vi "Magnet Idot Monitor.vi"(8 "Error In":errorcluster, 10 "Server port":u16=1002, 11 "Server address":string="192.168.1.100") -> (0 "Error Out":errorcluster)   [LabVIEW 2015]
uses:
  Libraries/Red Pitaya/Mode.ctl
  Libraries/Red Pitaya/Red Pitaya Parameters.ctl
  Libraries/Red Pitaya/RP Command.ctl
  Libraries/Utilities/Controls/Integrate channel.ctl
panel:
  out "Magnet current":waveform(dbl)(graph)
  in  "Controls":enum32{"Basic", "Advanced"}(tab)
  in  "Idot \ncalibration":dbl=-137722.0
  in  "Parameters":T1={"Ranges"=[1.12291, 20.0], "Output frequency 1"=50000.0, "Output frequency 2"=50000.0, "Trigger offset"=-2000000, "Post-trigger samples"=5767168, "Desimation rate"=64} {"Post-trigger samples" format="0x%x (%d)"; "Trigger offset" format="0x%x (%d)"; "Output frequency 2" format="%#_6p"; "Output frequency 1" format="%#_6p"; "Ranges" format="%#_12g"}
  out "CPU Temperature":dbl(slide)=48.847186279148 scale=0.0..100.0
  out "Current min/max":cluster{"Max":dbl, "Min":dbl}
  in  "Offset duration":dbl=0.95
  in  "Ch to \nintegrate":i32
  in  "Trigger pos acuracy":i32=2
  in  "Signal bits":i32=16
  in  "Read Temperature":bool=TRUE
  in  "Read trigger":bool=TRUE
  in  "Start server":bool
  in  "FPGA Logic":enum16{"Digitizer", "Fast Digitizer"}(ring)
  in  "Auto-save file":bool=TRUE
  in  "Samples to read":u64=67108864 format="0x%x (%d)"
  in  "Record":bool
  out "Server  output":string
  out "Temperature Chart":dbl(graph)=48.847186279148
  out "bytes written":i32=8
  in  "Status":bool
  out "Status response":u32=1
  out "element":u32
  in  "Status offset":u64=8 format="%x"
  out "Record start pos":u32=1
  out "x-y":u32=4294967295
  out "Phase increment 2":u64=1717987
  out "Phase increment 1":u64=1717987
  in  "Process Stop Button":bool
  in  "Read":bool
  in  "Read subset":bool
  out "Data File  Path":path
  out "Trigger state":bool
  in  "Trigger":bool
  in  "Arm":bool
  out "Phase  Graph":u32[](graph)
  in  "Mode":T2=enum."Digitizer"
  out "Waveform Graph":sgl[][](graph)
  in  "Stop Server":bool
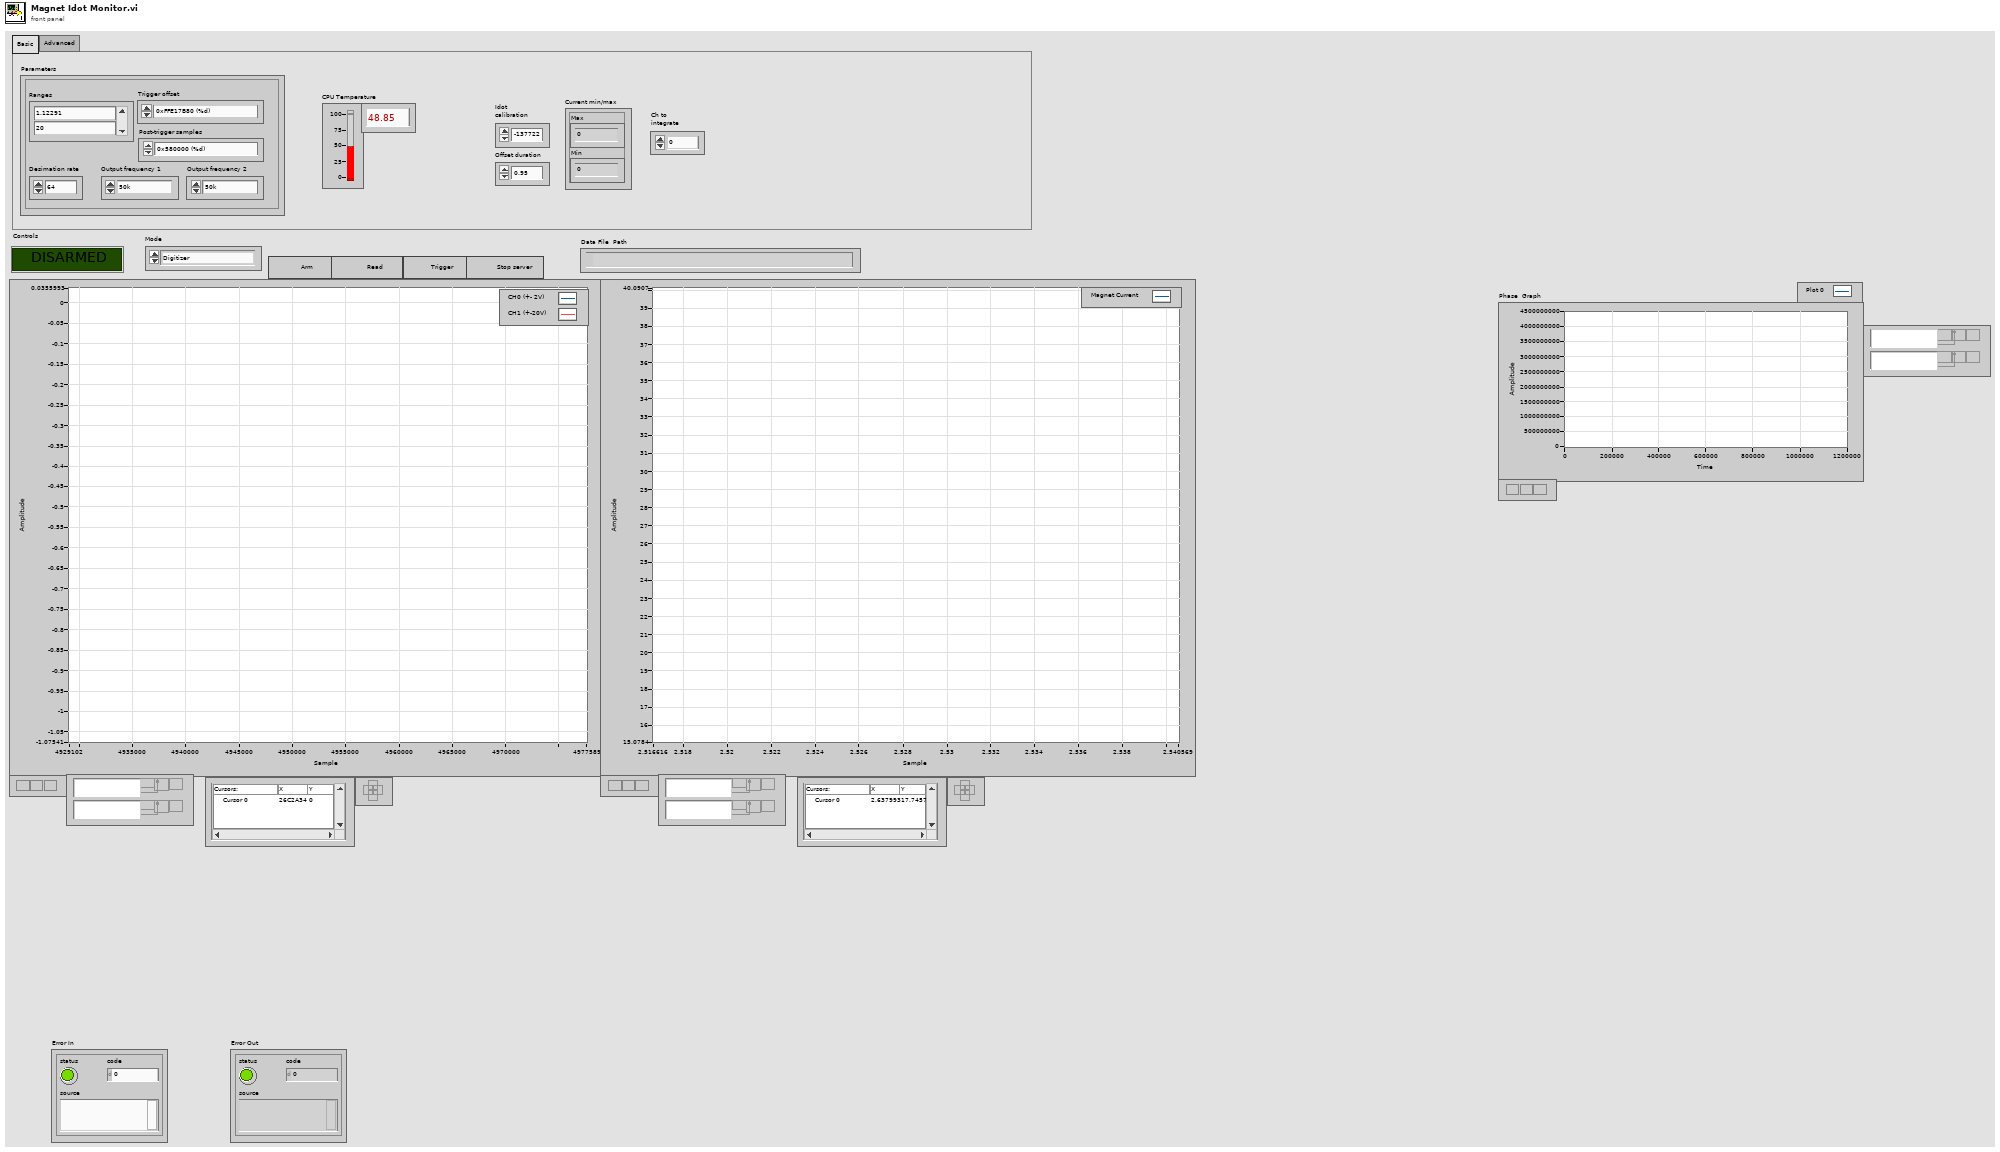
[diagram p1: front panel]
types:
  T1 = typedef "Red Pitaya Parameters.ctl" = cluster{"Ranges":dbl[], "Output frequency 1":dbl, "Output frequency 2":dbl, "Trigger offset":i32, "Post-trigger samples":u64, "Desimation rate":u64}
  T2 = typedef "Mode.ctl" = enum16{"Filter", "Lockin test", "Snapshot test", "Digitizer"}
  T3 = typedef "RP Command.ctl" = enum16{"Set frequency", "Arm and get data", "Stop server", "Get status", "Get temperature", "Set decimation", "Arm", "Software trigger", "Get whole buffer", "Get chunk", "System call", "Get config", "Set config"}
  T4 = typedef "Integrate channel.ctl" = cluster{"Channel":string, "Output name":string, "Factor":dbl, "Start time":dbl, "Duration":dbl}
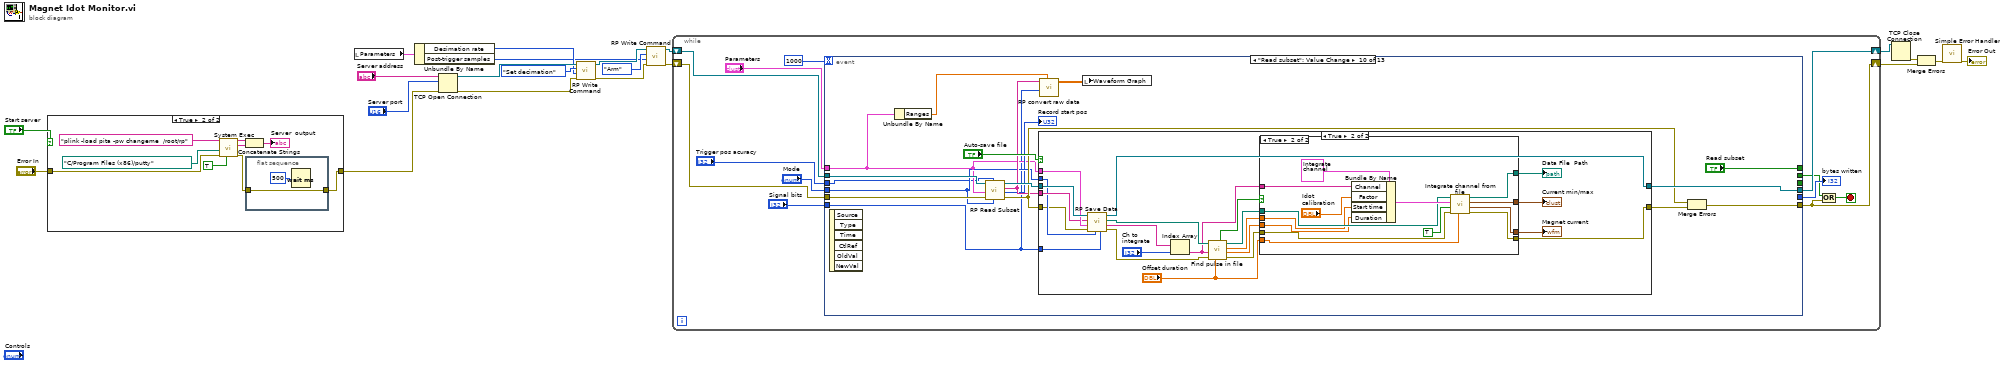
[diagram p0: block diagram]
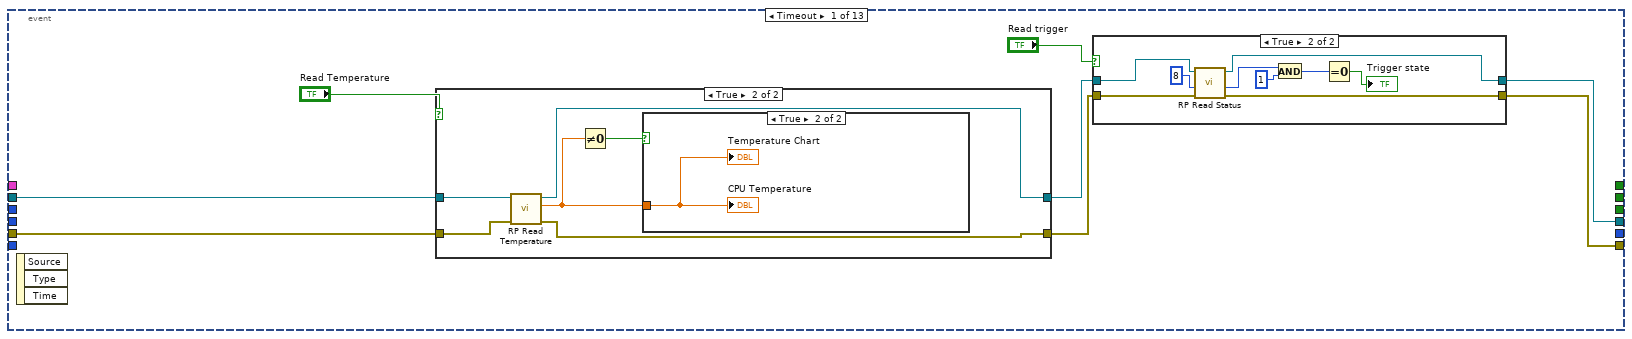
[diagram p3: hidden frame]
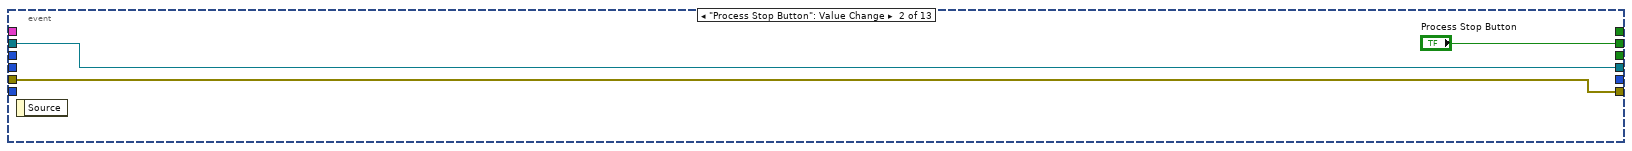
[diagram p7: hidden frame]
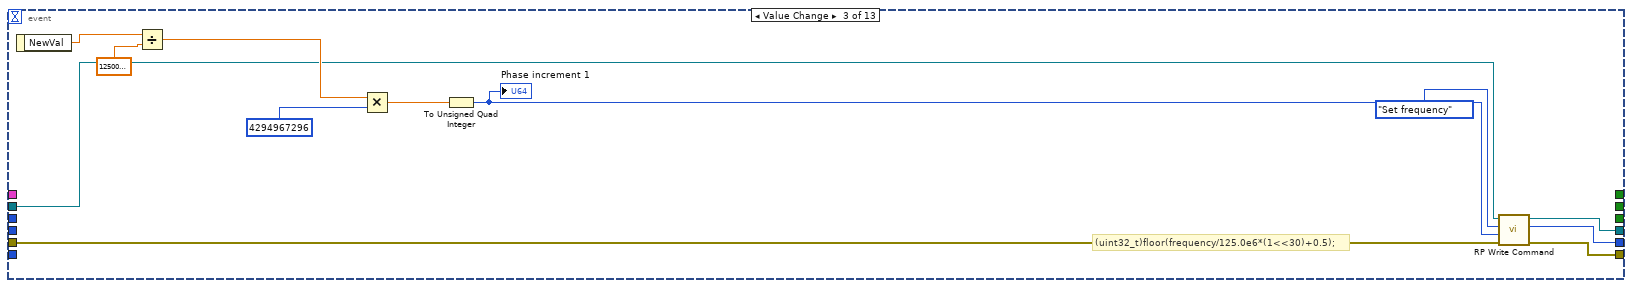
[diagram p8: hidden frame]
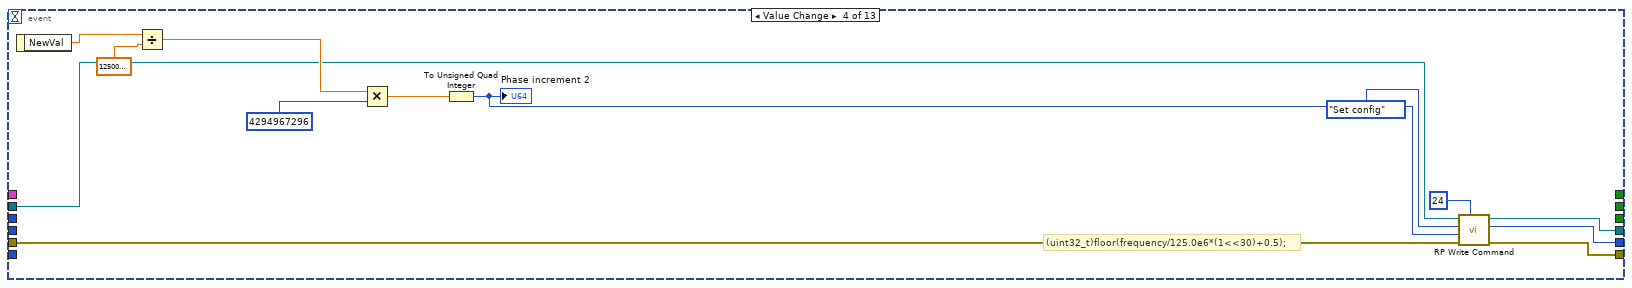
[diagram p9: hidden frame]
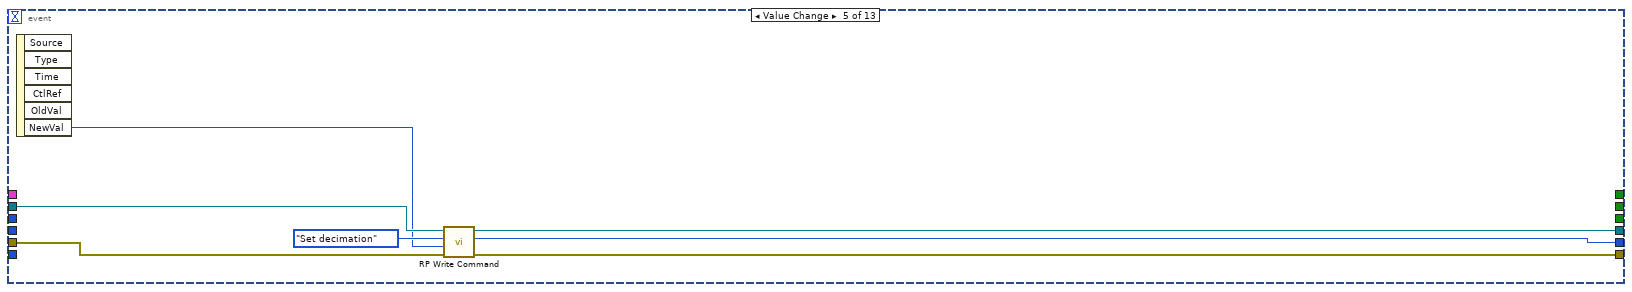
[diagram p10: hidden frame]
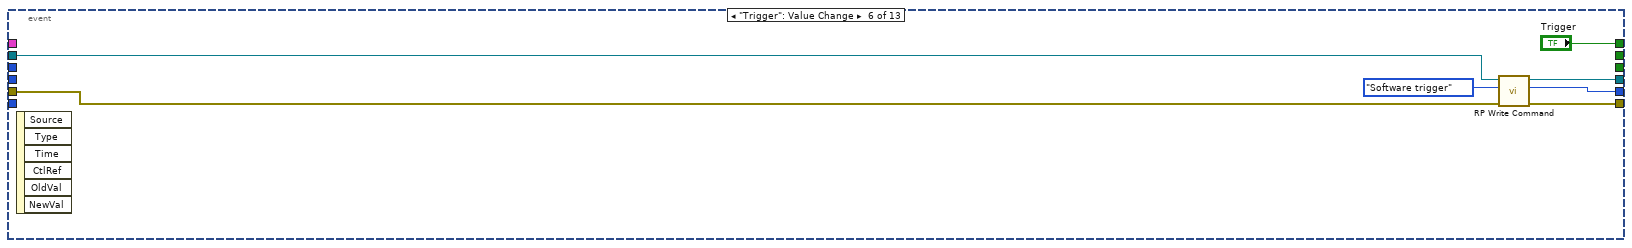
[diagram p11: hidden frame]
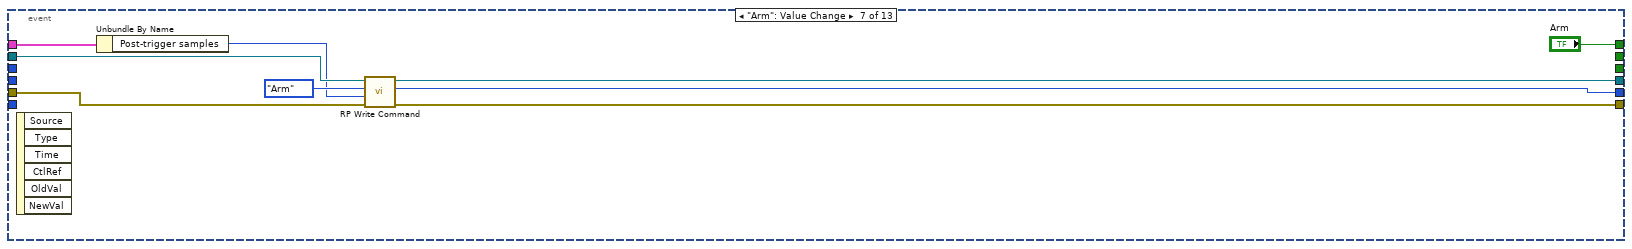
[diagram p12: hidden frame]
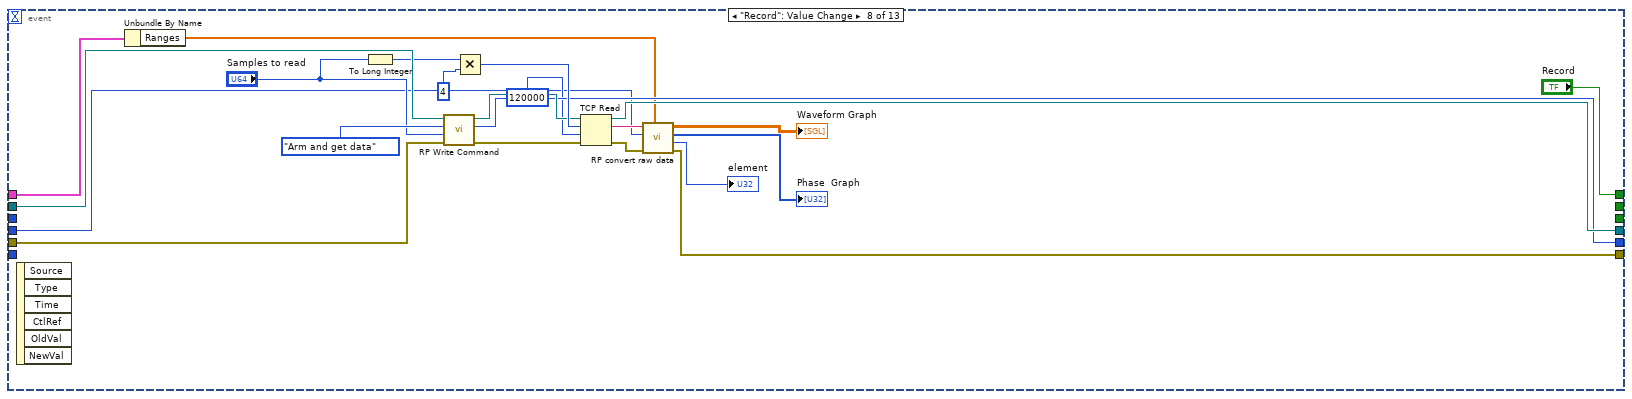
[diagram p13: hidden frame]
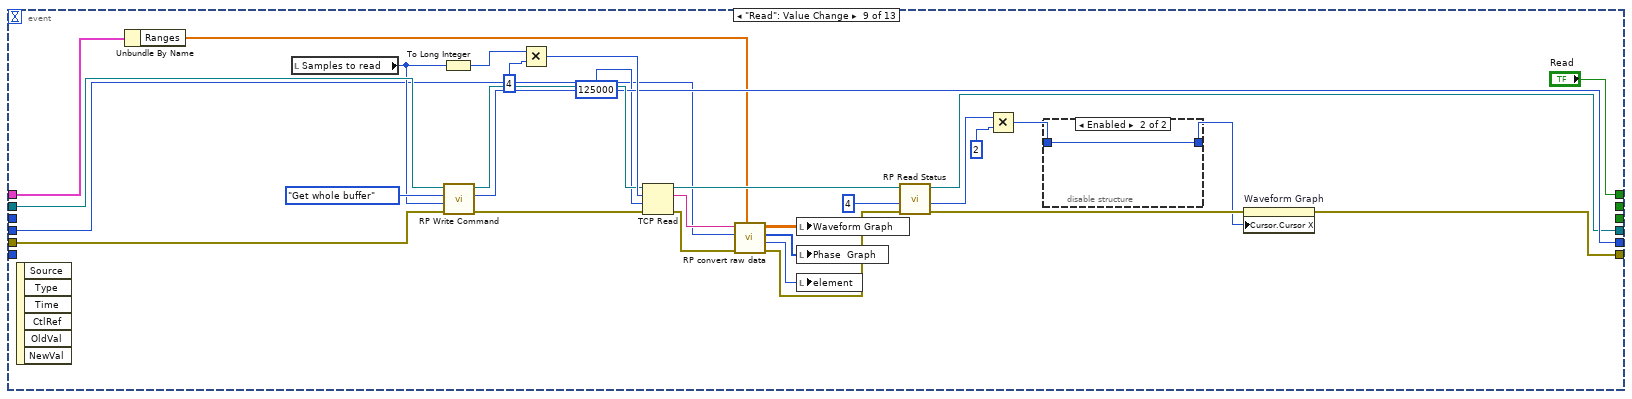
[diagram p14: hidden frame]
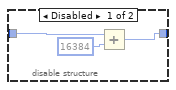
[diagram p15: hidden frame]
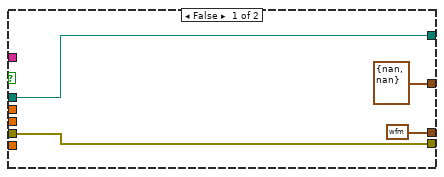
[diagram p17: hidden frame]
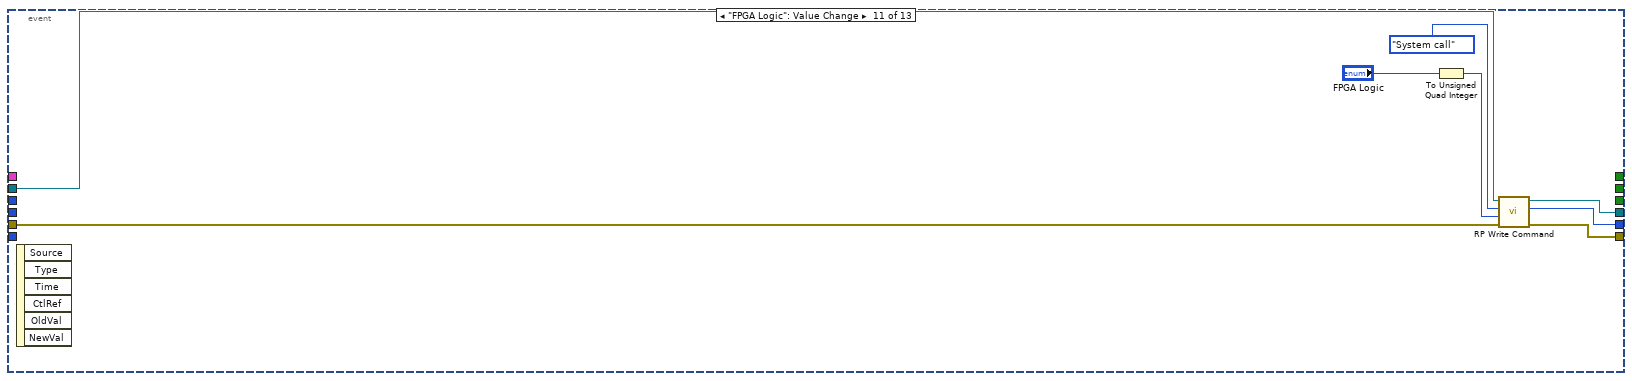
[diagram p18: hidden frame]
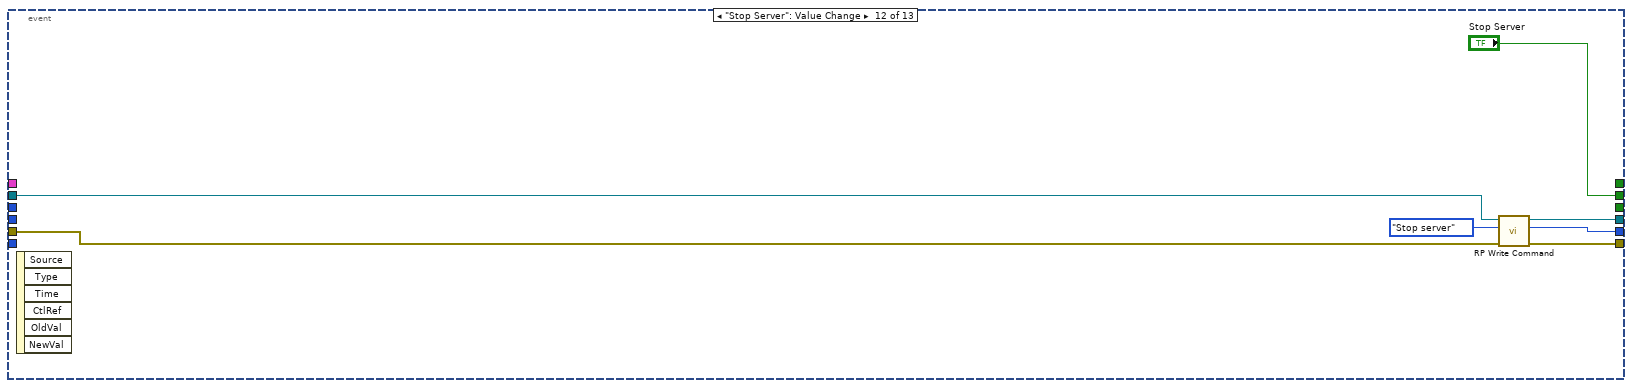
[diagram p19: hidden frame]
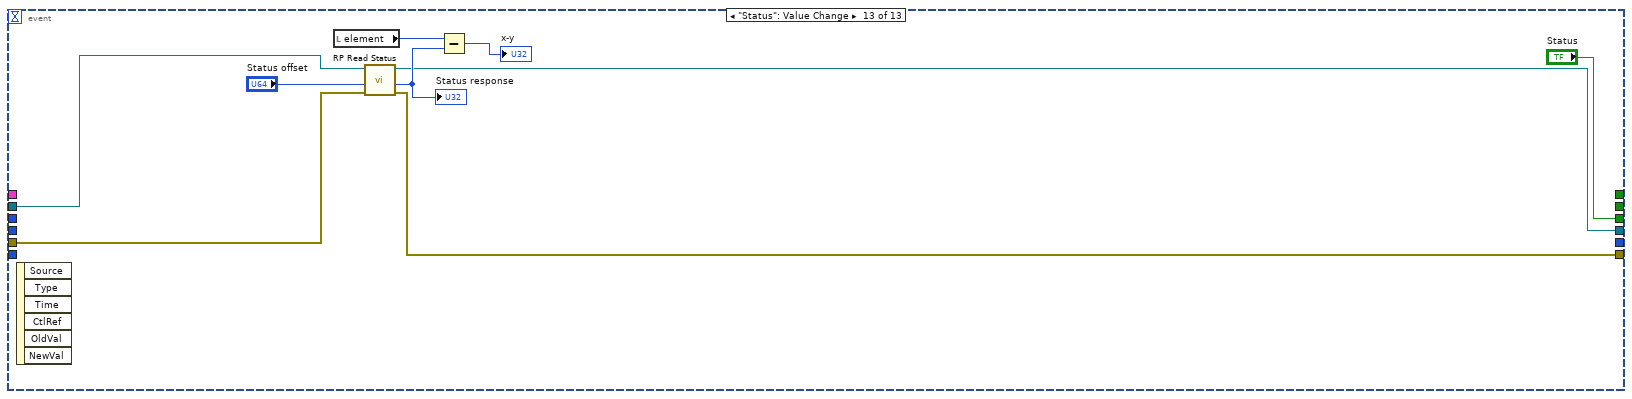
[diagram p20: hidden frame]
diagram:
  n1 = case shown="True" "Start server" {
    tunnel: [w22 w23] -> w11
    tunnel: "Error In" -> [w22 w25]
    frame False {
    }
    frame True {
      n2 = call <vilib>:"System Exec.vi"("run minimized? (F)"=TRUE, "error in (no error)"=w25, "working directory"=path "C:/Program Files (x86)/putty", "command line"="plink -load pita -pw changeme  /root/rp") -> ("error out"=w24:errorcluster, "standard error"=w27:string, "standard output"=w31:string)  [unwired: 4 in, 1 out]
      n3 = Concatenate Strings(w31, w27) -> (→"Server  output":string)
      n4 = flat-sequence {
        tunnel: w24 -> [w33]
        tunnel: [w33] -> w23
        frame #0 {
          n5 = Wait (ms)(milliseconds to wait=u32 500) -> ()  [unwired: 1 out]
        }
      }
    }
  }
  n6 = local read "Parameters"() -> (w8:T1)
  n7 = Unbundle By Name(w8) -> ("Desimation rate"=w7:u64, "Post-trigger samples"=w3:u64)
  n8 = TCP Open Connection(address="Server address", remote port or service name="Server port", error in (no error)=w11) -> (connection ID=w9:refnum<k5>, error out=w10:errorcluster)  [unwired: 2 in]
  n9 = call "RP Write Command.vi"("Error In"=w10, "Command payload"=w7, "Command number"=RP_Command."Set decimation", "connection ID"=w9) -> ("Error Out"=w4:errorcluster, "connection ID out"=w5:refnum<k5>)  [unwired: 5 in, 1 out]
  n10 = call "RP Write Command.vi"("Error In"=w4, "Command payload"=w3, "Command number"=RP_Command."Arm", "connection ID"=w5) -> ("Error Out"=w1:errorcluster, "connection ID out"=w2:refnum<k5>)  [unwired: 5 in, 1 out]
  n11 = while {
    shift-right: [w43] -> w17
    shift-left: w2 -> [w44]
    shift-right: [w41] -> w16
    shift-left: w1 -> [w45]
    stop <- w39 stop-if-true
    n12 = event shown="[9] \"Read subset\": Value Change" {
      selector: _ -> [_ _ _ _ _ _ _ _ _ _ _ _ _]
      dyn-events: _ -> [_ _ _ _ _ _ _ _ _ _ _ _ _]
      timeout: 1000 -> [_ _ _ _ _ _ _ _ _ _ _ _ _]
      tunnel: w45 -> [w51 w75 w84 w97 w108 w115 w124 w139 w171 w191 w247 w254 w260]
      tunnel: w44 -> [w52 w74 w83 w96 w107 w114 w123 w142 w174 w190 w246 w252 w256]
      tunnel: [w47 w75 w79 w92 w104 w111 w120 w130 w168 w195 w242 w251 w259] -> w41
      tunnel: [w46 w74 w80 w93 w105 w112 w121 w144 w164 w192 w241 w250 w257] -> w43
      tunnel: [_ "Process Stop Button" _ _ _ _ _ _ _ _ _ "Stop Server" _] -> w40
      tunnel: [_ _ _ _ _ _ _ _ _ _ _ _ "Status"] -> _
      tunnel: [_ _ w78 w91 w103 w110 w119 w137 w169 _ w240 w249 _] -> w42
      tunnel: [_ _ _ _ _ "Trigger" "Arm" "Record" "Read" "Read subset" _ _ _] -> _
      tunnel: "Mode" -> [_ _ _ _ _ _ _ w127 w149 w186 _ _ _]
      tunnel: "Parameters" -> [_ _ _ _ _ _ w117 w126 w148 w184 _ _ _]
      tunnel: "Signal bits" -> [_ _ _ _ _ _ _ _ _ w181 _ _ _]
      tunnel: "Trigger pos acuracy" -> [_ _ _ _ _ _ _ _ _ w182 _ _ _]
      event Timeout {
        n13 = event-data() -> ()  [unwired: 1 in, 3 out]
        n14 = case shown="True" "Read Temperature" {
          tunnel: w52 -> [w66 w71]
          tunnel: w51 -> [w65 w67]
          tunnel: [w66 w70] -> w49
          tunnel: [w65 w68] -> w48
          frame False {
          }
          frame True {
            n15 = call "RP Read Temperature.vi"("Error In"=w67, "connection ID"=w71) -> ("error out"=w68:errorcluster, "Thermometer"=w69:dbl, "connection ID out"=w70:refnum<k5>)  [unwired: 7 in]
            n16 = Not Equal To 0?(x=w69) -> (x != 0?=w72:bool)
            n17 = case shown="True" w72 {
              tunnel: w69 -> [_ w73]
              frame False {
              }
              frame True {
                "CPU Temperature" <- w73
                "Temperature Chart" <- w73
              }
            }
          }
        }
        n18 = case shown="True" "Read trigger" {
          tunnel: w49 -> [w54 w63]
          tunnel: w48 -> [w55 w64]
          tunnel: [w55 w59] -> w47
          tunnel: [w54 w56] -> w46
          frame False {
          }
          frame True {
            n19 = call "RP Read Status.vi"("Error In"=w64, "Status offset"=u64 8, "connection ID"=w63) -> ("Error Out"=w59:errorcluster, "Status response"=w61:u32, "connection ID out"=w56:refnum<k5>)  [unwired: 6 in]
            n20 = And(x=w61, y=u32 1) -> (x .and. y?=w58:u32)
            n21 = Equal To 0?(x=w58) -> (x = 0?=→"Trigger state":bool)
          }
        }
      }
      event "Process Stop Button": Value Change {
        n22 = event-data() -> ()  [unwired: 1 in, 1 out]
      }
      event Value Change {
        # "(uint32_t)floor(frequency/125.0e6*(1<<30)+0.5);"
        n23 = event-data() -> ("NewVal"=w77:dbl)  [unwired: 1 in]
        n24 = Divide(x=w77, y=125000000.0) -> (x/y=w86:dbl)
        n25 = Multiply(x=w86, y=i64 4294967296) -> (x*y=w85:dbl)
        n26 = To Unsigned Quad Integer(1:w85) -> (0:w81:u64)
        "Phase increment 1" <- w81
        n27 = call "RP Write Command.vi"("Error In"=w84, "Command payload"=w81, "Command number"=RP_Command."Set frequency", "connection ID"=w83) -> ("Error Out"=w79:errorcluster, "bytes written"=w78:i32, "connection ID out"=w80:refnum<k5>)  [unwired: 5 in]
      }
      event Value Change {
        # "(uint32_t)floor(frequency/125.0e6*(1<<30)+0.5);"
        n28 = event-data() -> ("NewVal"=w89:dbl)  [unwired: 1 in]
        n29 = Divide(x=w89, y=125000000.0) -> (x/y=w99:dbl)
        n30 = Multiply(x=w99, y=i64 4294967296) -> (x*y=w98:dbl)
        n31 = To Unsigned Quad Integer(1:w98) -> (0:w94:u64)
        "Phase increment 2" <- w94
        n32 = call "RP Write Command.vi"("Config offset"=u64 24, "Error In"=w97, "Command payload"=w94, "Command number"=RP_Command."Set config", "connection ID"=w96) -> ("Error Out"=w92:errorcluster, "bytes written"=w91:i32, "connection ID out"=w93:refnum<k5>)  [unwired: 4 in]
      }
      event Value Change {
        n33 = event-data() -> ("NewVal"=w102:u64)  [unwired: 1 in, 5 out]
        n34 = call "RP Write Command.vi"("Error In"=w108, "Command payload"=w102, "Command number"=RP_Command."Set decimation", "connection ID"=w107) -> ("Error Out"=w104:errorcluster, "bytes written"=w103:i32, "connection ID out"=w105:refnum<k5>)  [unwired: 5 in]
      }
      event "Trigger": Value Change {
        n35 = event-data() -> ()  [unwired: 1 in, 6 out]
        n36 = call "RP Write Command.vi"("Error In"=w115, "Command number"=RP_Command."Software trigger", "connection ID"=w114) -> ("Error Out"=w111:errorcluster, "bytes written"=w110:i32, "connection ID out"=w112:refnum<k5>)  [unwired: 6 in]
      }
      event "Arm": Value Change {
        n37 = event-data() -> ()  [unwired: 1 in, 6 out]
        n38 = Unbundle By Name(w117) -> ("Post-trigger samples"=w116:u64)
        n39 = call "RP Write Command.vi"("Error In"=w124, "Command payload"=w116, "Command number"=RP_Command."Arm", "connection ID"=w123) -> ("Error Out"=w120:errorcluster, "bytes written"=w119:i32, "connection ID out"=w121:refnum<k5>)  [unwired: 5 in]
      }
      event "Record": Value Change {
        n40 = event-data() -> ()  [unwired: 1 in, 6 out]
        n41 = Unbundle By Name(w126) -> ("Ranges"=w125:dbl[])
        n42 = To Long Integer(number="Samples to read") -> (32bit integer=w136:i32)
        n43 = call "RP Write Command.vi"("Error In"=w139, "Command payload"="Samples to read", "Command number"=RP_Command."Arm and get data", "connection ID"=w142) -> ("Error Out"=w138:errorcluster, "bytes written"=w137:i32, "connection ID out"=w140:refnum<k5>)  [unwired: 5 in]
        n44 = Multiply(x=w136, y=4) -> (x*y=w143:i32)
        n45 = TCP Read(connection ID=w140, bytes to read=w143, error in (no error)=w138, 9:120000 ("timeout ms (25000)")) -> (connection ID out=w144:refnum<k5>, data out=w133:string, error out=w131:errorcluster)  [unwired: 1 in]
        n46 = call "RP convert raw data.vi"("Max Volts"=w125, "Error In"=w131, "Format"=w127, "data stream"=w133) -> ("Error Out"=w130:errorcluster, "element"=→"element":u32, "phase out"=→"Phase  Graph":u32[], "data out"=→"Waveform Graph":sgl[][])  [unwired: 4 in]
      }
      event "Read": Value Change {
        n47 = event-data() -> ()  [unwired: 1 in, 6 out]
        n48 = Unbundle By Name(w148) -> ("Ranges"=w147:dbl[])
        n49 = local read "Samples to read"() -> (w163:u64)
        n50 = To Long Integer(number=w163) -> (32bit integer=w166:i32)
        n51 = call "RP Write Command.vi"("Error In"=w171, "Command payload"=w163, "Command number"=RP_Command."Get whole buffer", "connection ID"=w174) -> ("Error Out"=w170:errorcluster, "bytes written"=w169:i32, "connection ID out"=w172:refnum<k5>)  [unwired: 5 in]
        n52 = Multiply(x=w166, y=4) -> (x*y=w175:i32)
        n53 = TCP Read(connection ID=w172, bytes to read=w175, error in (no error)=w170, 9:125000 ("timeout ms (25000)")) -> (connection ID out=w165:refnum<k5>, data out=w161:string, error out=w151:errorcluster)  [unwired: 1 in]
        n54 = call "RP convert raw data.vi"("Max Volts"=w147, "Error In"=w151, "Format"=w149, "data stream"=w161) -> ("Error Out"=w150:errorcluster, "element"=w158:u32, "phase out"=w159:u32[], "data out"=w160:sgl[][])  [unwired: 4 in]
        n55 = local write "Waveform Graph"(w160) -> ()
        n56 = local write "Phase  Graph"(w159) -> ()
        n57 = local write "element"(w158) -> ()
        n58 = call "RP Read Status.vi"("Error In"=w150, "Status offset"=u64 4, "connection ID"=w165) -> ("Error Out"=w156:errorcluster, "Status response"=w155:u32, "connection ID out"=w164:refnum<k5>)  [unwired: 6 in]
        n59 = Multiply(x=w155, y=u32 2) -> (x*y=w153:u32)
        n60 = disable-structure shown="Enabled" {
          disable-tunnel: w153 -> [w179 w180]
          disable-tunnel: [w177 w180] -> w152
          frame Disabled {
            n61 = Add(x=w179, y=16384) -> (x+y=w177:u32)
          }
          frame Enabled {
          }
        }
        n62 = property on="Waveform Graph" class="WFGraph (strict)"(error in=w156, "Cursor.Cursor X"=w152) -> (error out=w168:errorcluster)  [unwired: 1 in, 1 out]
      }
      event "Read subset": Value Change {
        n63 = event-data() -> ()  [unwired: 1 in, 6 out]
        n64 = Unbundle By Name(w184) -> ("Ranges"=w183:dbl[])
        n65 = call "RP Read Subset.vi"("Mode"=w186, "Trigger pos acuracy"=w182, "Error In"=w191, "Parameters"=w184, "connection ID"=w190) -> ("Error Out"=w188:errorcluster, "Record start pos"=→"Record start pos":u32, "Data stream"=w187:string, "connection ID out"=w189:refnum<k5>)  [unwired: 3 in]
        n66 = case shown="True" "Auto-save file" {
          tunnel: w188 -> [w199 w216]
          tunnel: w187 -> [_ w219]
          tunnel: [w199 w213] -> w194
          tunnel: w189 -> [w198 w221]
          tunnel: [w198 w217] -> w192
          tunnel: w184 -> [_ w220]
          tunnel: w186 -> [_ w218]
          tunnel: w181 -> [_ w215]
          frame False {
          }
          frame True {
            n67 = call "RP Save Data.vi"("Signal bits"=w215, "Mode"=w218, "Error In"=w216, "Parameters"=w220, "Data stream"=w219, "connection ID"=w221) -> ("Error Out"=w206:errorcluster, "Channel names"=w212:string[], "Data File  Path"=w207:path, "connection ID out"=w217:refnum<k5>)  [unwired: 2 in]
            n68 = Index Array(array=w212, index="Ch to \nintegrate") -> (element=w204:string)
            n69 = call "Find pulse in file.vi"("Offset duration"="Offset duration", "Error In"=w206, "Channel"=w204, "File Path Control"=w207) -> ("Error Out"=w205:errorcluster, "duration"=w201:dbl, "Start time"=w202:dbl, "File Path out"=w208:path, "Found"=w203:bool)  [unwired: 3 in]
            n70 = case shown="True" w203 {
              tunnel: [w225 w239] -> w214
              tunnel: [w222 w238] -> w213
              tunnel: "Offset duration" -> [_ w235]
              tunnel: [cluster{"Max":dbl, "Min":dbl} {"Max"=nan, "Min"=nan} ("Min max") w234] -> w211
              tunnel: [waveform(dbl) {"t0"=timestamp(0 s since 1904-01-01), "dt"=1.0, "Y"=[]} ("Integrated Waveform") w233] -> w210
              tunnel: w208 -> [w225 w232]
              tunnel: w205 -> [w222 w231]
              tunnel: w204 -> [_ w230]
              tunnel: w202 -> [_ w229]
              tunnel: w201 -> [_ w228]
              frame False {
              }
              frame True {
                n71 = Bundle By Name(cluster=T4 {"Channel"="", "Output name"="Magnet Current", "Factor"=1.0, "Start time"=0.0, "Duration"=0.0} ("Integration settings"), "Channel"=w230, "Factor"="Idot \ncalibration", "Start time"=w229, "Duration"=w228) -> (w237:T4)
                n72 = call "Integrate channel from file.vi"("Offset duration"=w235, "Error In"=w231, "Save data"=TRUE, "Integration settings"=w237, "File Path Control"=w232) -> ("Error Out"=w238:errorcluster, "Integrated Waveform"=w233:waveform(dbl), "Min max"=w234:cluster{"Max":dbl, "Min":dbl}, "File Path out"=w239:path)  [unwired: 3 in]
              }
            }
            "Data File  Path" <- w214
            "Current min/max" <- w211
            "Magnet current" <- w210
          }
        }
        n73 = call "RP convert raw data.vi"("Max Volts"=w183, "Signal bits"=w181, "data stream"=w187) -> ("data out"=w193:sgl[][])  [unwired: 5 in, 3 out]
        n74 = local write "Waveform Graph"(w193) -> ()
        n75 = Merge Errors(w188, w194) -> (w195:errorcluster)
      }
      event "FPGA Logic": Value Change {
        n76 = event-data() -> ()  [unwired: 1 in, 6 out]
        n77 = To Unsigned Quad Integer(1:"FPGA Logic") -> (0:w244:u64)
        n78 = call "RP Write Command.vi"("Error In"=w247, "Command payload"=w244, "Command number"=RP_Command."System call", "connection ID"=w246) -> ("Error Out"=w242:errorcluster, "bytes written"=w240:i32, "connection ID out"=w241:refnum<k5>)  [unwired: 5 in]
      }
      event "Stop Server": Value Change {
        n79 = event-data() -> ()  [unwired: 1 in, 6 out]
        n80 = call "RP Write Command.vi"("Error In"=w254, "Command number"=RP_Command."Stop server", "connection ID"=w252) -> ("Error Out"=w251:errorcluster, "bytes written"=w249:i32, "connection ID out"=w250:refnum<k5>)  [unwired: 6 in]
      }
      event "Status": Value Change {
        n81 = event-data() -> ()  [unwired: 1 in, 6 out]
        n82 = local read "element"() -> (w262:u32)
        n83 = call "RP Read Status.vi"("Error In"=w260, "Status offset"="Status offset", "connection ID"=w256) -> ("Error Out"=w259:errorcluster, "Status response"=w258:u32, "connection ID out"=w257:refnum<k5>)  [unwired: 6 in]
        "Status response" <- w258
        n84 = Subtract(x=w262, y=w258) -> (x-y=→"x-y":u32)
      }
    }
    "bytes written" <- w42
    n85 = Or(x=w40, y=w41) -> (x .or. y?=w39:bool)
  }
  n86 = TCP Close Connection(connection ID=w17) -> (error out=w19:errorcluster)  [unwired: 2 in, 1 out]
  n87 = Merge Errors(w19, w16) -> (w18:errorcluster)
  n88 = call <vilib>:"Simple Error Handler.vi"("error in (no error)"=w18) -> ("error out"=→"Error Out":errorcluster)  [unwired: 4 in, 4 out]
